vi "Call DQMH Request and Wait for Reply VI QD.vi"(8 "error in (no error)":errorcluster, 11 "Request VI in":refnum<vi>) -> (0 "error out":errorcluster, 2 "Is Request and Wait for Reply":bool, 3 "Request VI out":refnum<vi>)   [LabVIEW 2017]
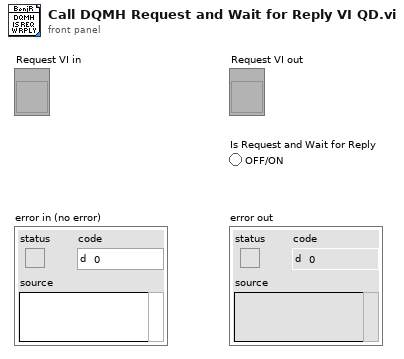
[diagram p1: front panel]
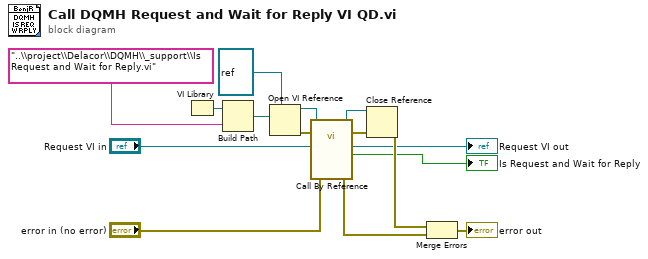
[diagram p0: block diagram]
diagram:
  n1 = VI Library() -> (path=w11:path)
  n2 = Build Path(base path=w11, name or relative path="..\\project\\Delacor\\DQMH\\_support\\Is Request and Wait for Reply.vi") -> (appended path=w10:path)
  n3 = Open VI Reference(type specifier VI Refnum (for type only)=refnum<vi> refnum, vi path=w10) -> (vi reference=w15:refnum<vi>, error out=w5:errorcluster)  [unwired: 4 in]
  n4 = call-by-ref "?"(reference=w15, error in=w5, 8:"error in (no error)"="error in (no error)", "Request VI in"="Request VI in") -> (reference out=w13:refnum<vi>, error out=w14:errorcluster, 0:"error out"=w9:errorcluster, "Is Request"=→"Is Request and Wait for Reply":bool, "Request VI out"=→"Request VI out":refnum<vi>)  [unwired: 7 in]
  n5 = Close Reference(reference=w13, error in (no error)=w14) -> (error out=w8:errorcluster)
  n6 = Merge Errors(w8, w9) -> (→"error out":errorcluster)
